vi "Main.vi"(10 "Monedas Sub Panel":refnum<vi>, 11 "Module Admin":refnum<class "Delacor_lib_QMH_Module Admin.lvclass">) -> ()   [LabVIEW 2020, in "Monedas.lvlib"]
doc: "This template is based off of the Queued Message Handler design pattern and the Queued Message Handler project template that ships with LabVIEW.\n\nThe main difference is that the queue is private to this module and communication between modules is performed via Broadcast and Request events.\n\nRequest events are wrapped in public API methods and are handled in the Event Handling Loop (EHL) of this VI. Any module can register for Broadcast events sent by this module. The EHL generates messages based on user interface actions.\n\nThe Message Handling Loop (MHL) processes messages generated by the EHL, or by other messages. The messages are string values, so new messages can be added easily to the Message Cases case structure in the MHL. Each message cluster can also provide an optional value for Message Data, which is a variant that can be converted to whatever message-specific data is required.\n_____\nBased on Delacor QMH Project Template 5.0.0.82."
uses:
  Monedas.lvlib
  <vilib>/Delacor/Delacor QMH/Libraries/Module Admin_class/Delacor_lib_QMH_Module Admin.lvclass
  Module Data--cluster.ctl
  Stop Argument--cluster.ctl
  <vilib>/Delacor/Delacor QMH/Libraries/Message Queue_class/Delacor_lib_QMH_Message Queue.lvclass/Delacor_lib_QMH_Message Queue.ctl
  Set Monedas Argument--cluster.ctl
  Producto Comprado Argument--cluster.ctl
  <vilib>/Delacor/Delacor QMH/Libraries/Module Admin_class/Delacor_lib_QMH_Module Admin.lvclass/Delacor_lib_QMH_Module Admin.ctl
  <vilib>/Delacor/Delacor QMH/Libraries/Message Queue_class/Delacor_lib_QMH_Enqueue Message (Single).vi
  <vilib>/Delacor/Delacor QMH/Libraries/Module Admin_class/Delacor_lib_QMH_Get External Launch.vi
  <vilib>/Utility/error.llb/Error Cluster From Error Code.vi
  <vilib>/ErrorRing/Error Ring.xnode
  <vilib>/Delacor/Delacor QMH/Libraries/Message Queue_class/Delacor_lib_QMH_Message Queue.lvclass
  Mensajes/Mensajes.lvlib
  Productos/Productos.lvlib
panel:
  in  "Monedas":T1
  out "error out":errorcluster
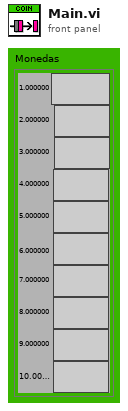
[diagram p1: front panel]
types:
  T1 = cluster{"Moneda 1":bool, "Moneda 2":bool, "Moneda 3":bool, "Moneda 4":bool, "Moneda 5":bool, "Moneda 6":bool, "Moneda 7":bool, "Moneda 8":bool, "Moneda 9":bool, "Moneda 10":bool}
  T2 = typedef "Monedas.lvlib/Request Events--cluster.ctl" = cluster{"Stop Module":refnum<user-event>, "Show Panel":refnum<user-event>, "Hide Panel":refnum<user-event>, "Get Module Execution Status":refnum<user-event>, "Show Diagram":refnum<user-event>, "Set Monedas":refnum<user-event>, "Producto Comprado":refnum<user-event>}
  T3 = typedef "Monedas.lvlib/Module Data--cluster.ctl" = cluster{"Status":string, "Array":cluster{"Numeric":dbl, "Boolean":bool}[], "Crédito":dbl}
  T4 = enum32{"invalid lock state", "Not Locked", "Locked (No Password)", "Password-protected"}
  T5 = typedef "Monedas.lvlib/Stop Argument--cluster.ctl" = cluster{"Origin":string, "Exit via Stop Module Req?":bool, "Wait for Module to stop?":bool}
  T6 = typedef "Monedas.lvlib/Set Monedas Argument--cluster.ctl" = cluster{"Monedas":cluster{"Numeric":dbl, "Boolean":bool}[]}
  T7 = typedef "Monedas.lvlib/Producto Comprado Argument--cluster.ctl" = cluster{"Numeric":dbl}
  T8 = enum32{"Invalid", "Standard", "Closed", "Hidden", "Minimized", "Maximized"}
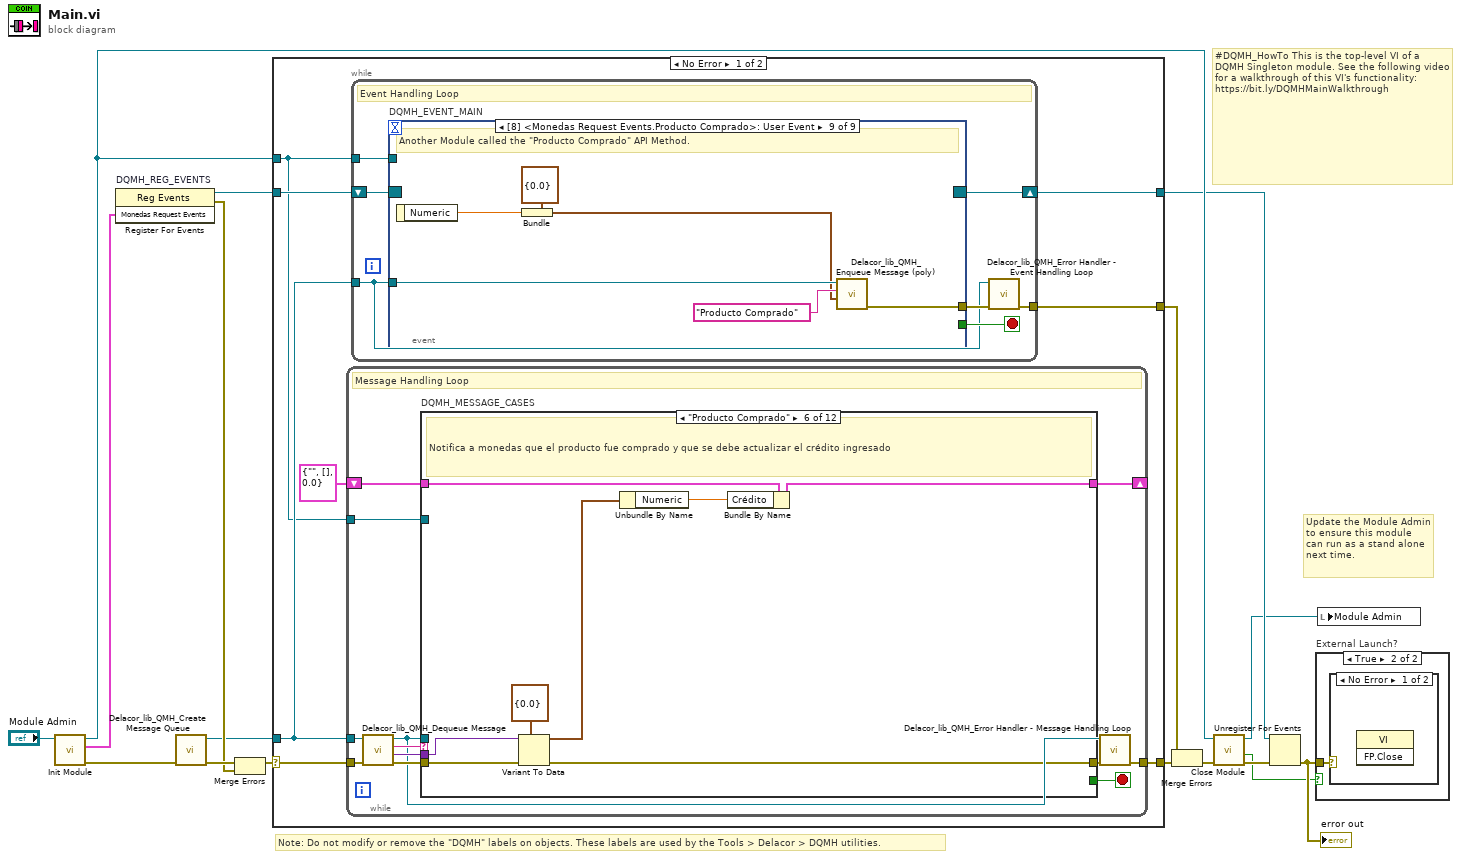
[diagram p0: block diagram]
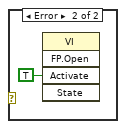
[diagram p3: hidden frame]
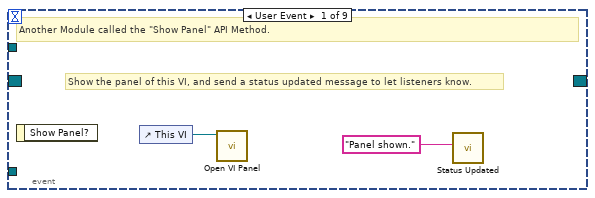
[diagram p4: hidden frame]
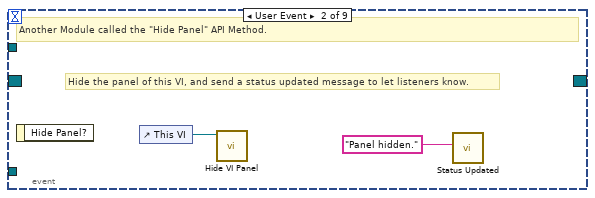
[diagram p5: hidden frame]
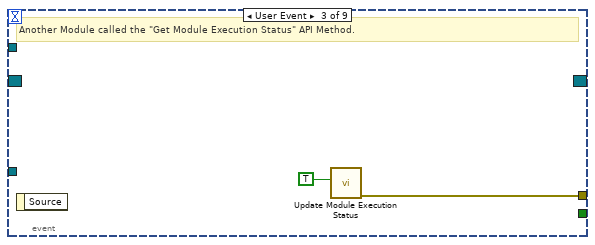
[diagram p6: hidden frame]
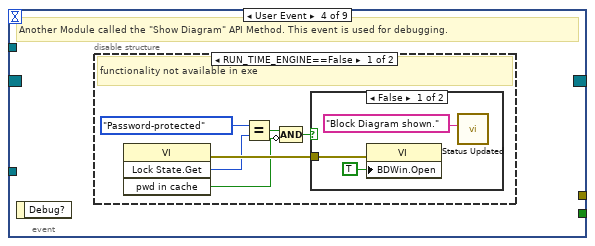
[diagram p7: hidden frame]
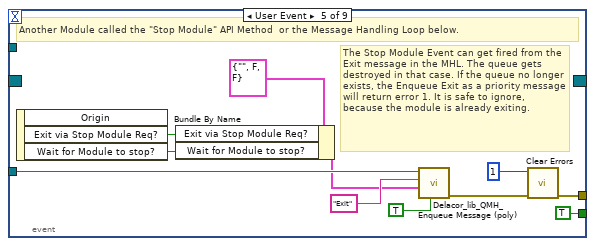
[diagram p10: hidden frame]
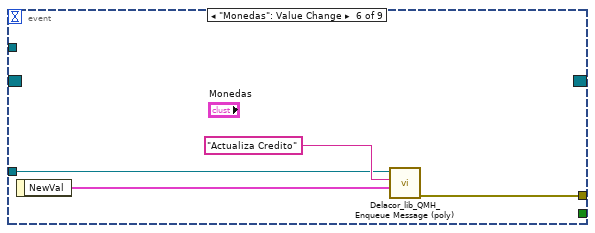
[diagram p11: hidden frame]
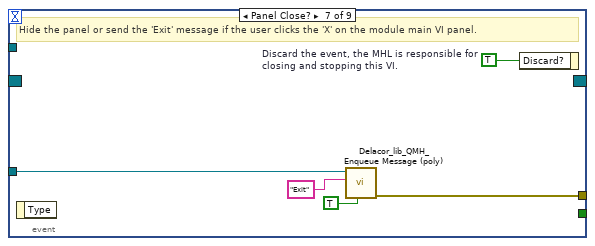
[diagram p12: hidden frame]
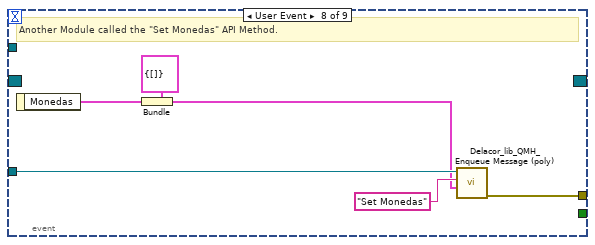
[diagram p13: hidden frame]
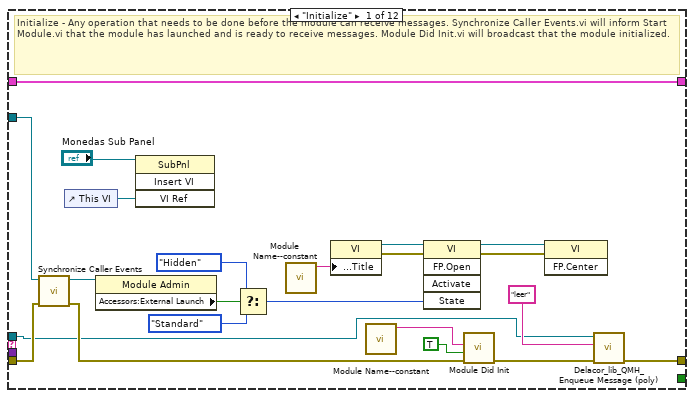
[diagram p14: hidden frame]
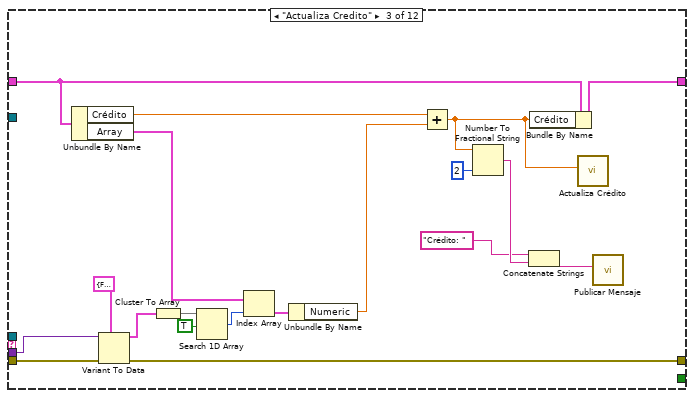
[diagram p16: hidden frame]
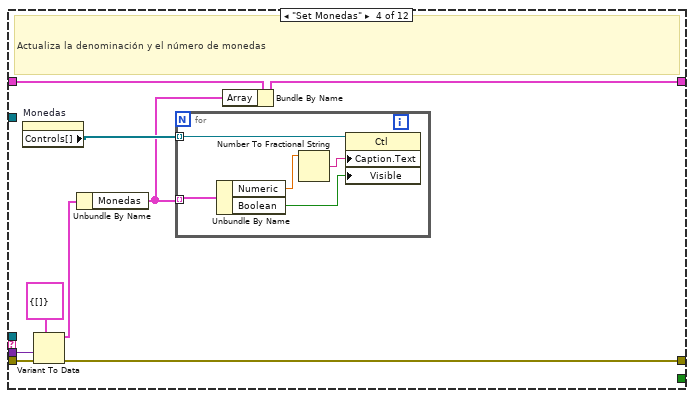
[diagram p17: hidden frame]
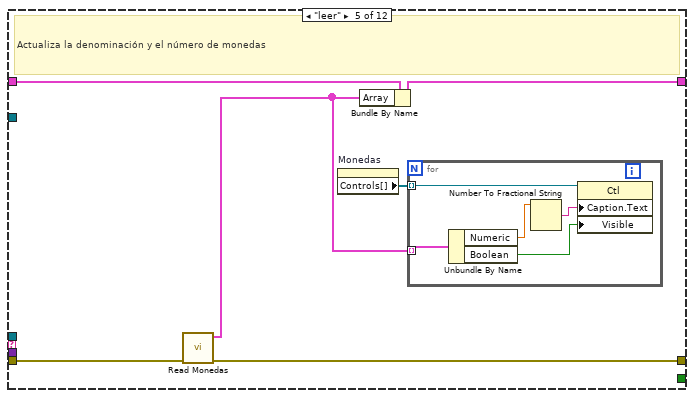
[diagram p18: hidden frame]
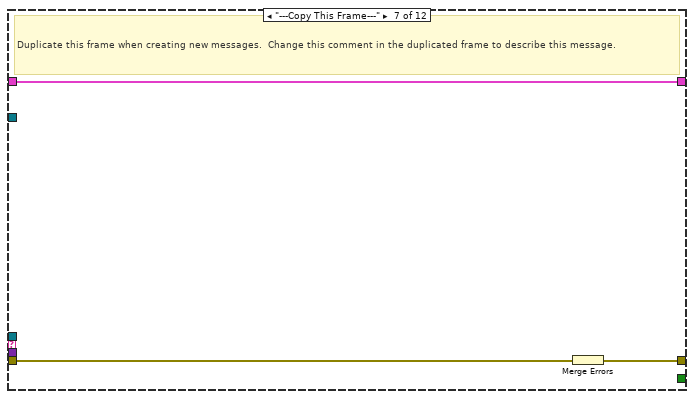
[diagram p19: hidden frame]
diagram:
  # "#DQMH_HowTo This is the top-level VI of a DQMH Singleton module. See the following video for a walkthrough of this VI's functionality: https://bit.ly/DQMHMainWalkthrough"
  # "Note: Do not modify or remove the \"DQMH\" labels on objects. These labels are used by the Tools > Delacor > DQMH utilities."
  # "Update the Module Admin to ensure this module can run as a stand alone next time."
  n1 = call "Init Module.vi"("Singleton Module Admin in"="Module Admin") -> ("error out"=w16:errorcluster, "Monedas Request Events"=w5:T2, "Singleton Module Admin out"=w8:refnum<class "Delacor_lib_QMH_Module Admin.lvclass">)  [unwired: 8 in]
  n2 = register-events "DQMH_REG_EVENTS"(w5) -> (reference out=w6:refnum<event-registration>, error out=w9:errorcluster)  [unwired: 2 in]
  n3 = call <vilib>:"Delacor_lib_QMH_Create Message Queue.vi"("error in (no error)"=w16) -> ("error out"=w11:errorcluster, "Message Queue"=w4:refnum<class "Delacor_lib_QMH_Message Queue.lvclass">)  [unwired: 9 in]
  n4 = Merge Errors(w11, w9) -> (w10:errorcluster)
  n5 = case shown="No Error" w10 {
    selector: w10 -> [w23 w233]
    tunnel: [w25 w232] -> w17
    tunnel: [w22 w238] -> w7
    tunnel: w6 -> [w20 w238]
    tunnel: w4 -> [w19 w231]
    tunnel: [w24 _] -> w14
    tunnel: w8 -> [w18 w234]
    frame No Error {
      n6 = while {
        tunnel: w19 -> [w82]
        shift-right: [w86] -> _
        shift-left: T3 {"Status"="", "Array"=[], "Crédito"=0.0} ("Data Cluster") -> [w87]
        tunnel: w23 -> [w90]
        tunnel: [w88] -> w25
        tunnel: w18 -> [w80]
        stop <- w85 stop-if-true
        # "Message Handling Loop"
        n7 = call-dynamic "Delacor_lib_QMH_Dequeue Message.vi"("error in (no error)"=w90, "Message Queue in"=w82) -> ("error out"=w89:errorcluster, "Message Data"=w83:variant, "Message"=w84:string, "Message Queue out"=w81:refnum<class "Delacor_lib_QMH_Message Queue.lvclass">)  [unwired: 6 in]
        n8 = case "DQMH_MESSAGE_CASES" shown="\"Producto Comprado\"" w84 {
          selector: w84 -> [_ _ _ _ _ _ _ _ _ _ _ w218]
          tunnel: w81 -> [w92 _ _ _ _ _ _ _ _ w188 w210 _]
          tunnel: w89 -> [w111 w115 w134 w143 w152 w167 w170 w172 w177 w195 w216 w220]
          tunnel: [w93 w115 w121 w135 w153 w165 w169 w172 w176 w191 w213 w221] -> w91
          tunnel: w87 -> [w101 w114 w127 w142 w154 w166 w168 w171 w174 w190 w209 w219]
          tunnel: [w101 w114 w124 w138 w151 w161 w168 w171 w174 w190 w209 w219] -> w86
          tunnel: [_ _ _ _ _ _ _ _ _ _ w208 _] -> w85
          tunnel: w83 -> [_ _ w133 w141 _ w164 _ _ _ w189 w207 _]
          tunnel: w80 -> [w102 _ _ _ _ _ _ _ _ w187 w202 _]
          frame "Initialize" {
            # "Initialize - Any operation that needs to be done before the module can receive messages. Synchronize Caller Events.vi will inform Start Module.vi that the module has launched and is ready to receive messages. Module Did Init.vi will broadcast that the module initialized."
            n9 = call "Synchronize Caller Events.vi"("error in (no error)"=w111, "Singleton Module Admin in"=w102) -> ("error out"=w110:errorcluster, "Singleton Module Admin out"=w98:refnum<class "Delacor_lib_QMH_Module Admin.lvclass">)  [unwired: 8 in]
            n10 = control-ref of="This VI"() -> (w96:refnum<vi>)
            n11 = property class="Module Admin"(reference=w98) -> ("Accessors:External Launch"=w106:bool)  [unwired: 1 in, 2 out]
            n12 = invoke class="SubPnl" method="Insert VI"(reference="Monedas Sub Panel", "VI Ref"=w96) -> ()  [unwired: 2 in, 4 out]
            n13 = Select(t=T8."Hidden" ("State"), s=w106, f=T8."Standard" ("State")) -> (s? t:f=w103:T8)
            n14 = call "Module Name--constant.vi"() -> ("Module Name"=w109:string)  [unwired: 11 in]
            n15 = property class="VI"("Front Panel.Title"=w109) -> (reference out=w108:refnum<vi>, error out=w113:errorcluster)  [unwired: 2 in]
            n16 = call "Module Name--constant.vi"() -> ("Module Name"=w99:string)  [unwired: 11 in]
            n17 = invoke class="VI" method="FP.Open"(reference=w108, error in=w113, "State"=w103) -> (reference out=w107:refnum<vi>, error out=w112:errorcluster)  [unwired: 2 in, 3 out]
            n18 = call "Module Did Init.vi"("error in (no error)"=w110, "Initialized?"=TRUE, "Origin"=w99) -> ("error out"=w94:errorcluster)  [unwired: 8 in]
            n19 = invoke class="VI" method="FP.Center"(reference=w107, error in=w112) -> ()  [unwired: 1 in, 3 out]
            n20 = call-poly <vilib>:"Delacor_lib_QMH_Enqueue Message (poly).vi"("error in (no error)"=w94, "Message"="leer", "Message Queue in"=w92) -> ("error out"=w93:errorcluster)  [unwired: 7 in, 1 out]
          }
          frame "--- Module Specific ---" {
            # "Separator -- The following cases handle messages specific to this Module."
          }
          frame "Actualiza Credito" {
            n21 = Unbundle By Name(w127) -> ("Crédito"=w122:dbl, "Array"=w126:cluster{"Numeric":dbl, "Boolean":bool}[])
            n22 = Variant To Data(error in=w134, type=T1 {"Moneda 1"=FALSE, "Moneda 2"=FALSE, "Moneda 3"=FALSE, "Moneda 4"=FALSE, "Moneda 5"=FALSE, "Moneda 6"=FALSE, "Moneda 7"=FALSE, "Moneda 8"=FALSE, "Moneda 9"=FALSE, "Moneda 10"=FALSE} ("Monedas"), Variant=w133) -> (data=w129:T1, error out=w121:errorcluster)
            n23 = Cluster To Array(cluster=w129) -> (array=w132:bool[])
            n24 = Search 1D Array(1D array=w132, element=TRUE) -> (index of element=w128:i32)  [unwired: 1 in]
            n25 = Index Array(array=w126, index=w128) -> (element=w125:cluster{"Numeric":dbl, "Boolean":bool})
            n26 = Unbundle By Name(w125) -> ("Numeric"=w123:dbl)
            n27 = Add(x=w122, y=w123) -> (x+y=w116:dbl)
            n28 = Number To Fractional String(number=w116, precision (6)=i16 2) -> (F-format string=w119:string)  [unwired: 2 in]
            n29 = Concatenate Strings("Crédito: " ("string"), w119) -> (w118:string)
            n30 = Bundle By Name(cluster=w127, "Crédito"=w116) -> (w124:T3)
            n31 = call "Actualiza Crédito.vi"("Crédito"=w116) -> ()  [unwired: 10 in, 1 out]
            n32 = call "Publicar Mensaje.vi"("Mensaje"=w118) -> ()  [unwired: 10 in, 1 out]
          }
          frame "Set Monedas" {
            # "Actualiza la denominación y el número de monedas"
            n33 = property on="Monedas" class="Clust"() -> ("Controls[]"=w137:refnum<vi>[])  [unwired: 2 in, 2 out]
            n34 = Variant To Data(error in=w143, type=T6 {"Monedas"=[]} ("Set Monedas Argument"), Variant=w141) -> (data=w139:T6, error out=w135:errorcluster)
            n35 = Unbundle By Name(w139) -> ("Monedas"=w136:cluster{"Numeric":dbl, "Boolean":bool}[])
            n36 = for {
              tunnel: w137 -> [w148] mode=indexing
              tunnel: w136 -> [w144] mode=indexing
              n37 = Unbundle By Name(w144) -> ("Numeric"=w146:dbl, "Boolean"=w145:bool)
              n38 = Number To Fractional String(number=w146) -> (F-format string=w147:string)  [unwired: 3 in]
              n39 = property class="Ctl"(reference=w148, "Caption.Text"=w147, "Visible"=w145) -> ()  [unwired: 1 in, 2 out]
            }
            n40 = Bundle By Name(cluster=w142, "Array"=w136) -> (w138:T3)
          }
          frame "leer" {
            # "Actualiza la denominación y el número de monedas"
            n41 = call "Read Monedas.vi"("error in (no error)"=w152) -> ("error out"=w153:errorcluster, "Array"=w150:cluster{"Numeric":dbl, "Boolean":bool}[])  [unwired: 9 in]
            n42 = property on="Monedas" class="Clust"() -> ("Controls[]"=w149:refnum<vi>[])  [unwired: 2 in, 2 out]
            n43 = Bundle By Name(cluster=w154, "Array"=w150) -> (w151:T3)
            n44 = for {
              tunnel: w149 -> [w159] mode=indexing
              tunnel: w150 -> [w157] mode=indexing
              n45 = Unbundle By Name(w157) -> ("Numeric"=w156:dbl, "Boolean"=w155:bool)
              n46 = Number To Fractional String(number=w156) -> (F-format string=w158:string)  [unwired: 3 in]
              n47 = property class="Ctl"(reference=w159, "Caption.Text"=w158, "Visible"=w155) -> ()  [unwired: 1 in, 2 out]
            }
          }
          frame "Producto Comprado" {
            # "Notifica a monedas que el producto fue comprado y que se debe actualizar el crédito ingresado"
            n48 = Variant To Data(error in=w167, type=T7 {"Numeric"=0.0} ("Producto Comprado Argument"), Variant=w164) -> (data=w162:T7, error out=w165:errorcluster)
            n49 = Unbundle By Name(w162) -> ("Numeric"=w160:dbl)
            n50 = Bundle By Name(cluster=w166, "Crédito"=w160) -> (w161:T3)
          }
          frame "---Copy This Frame---" {
            # "Duplicate this frame when creating new messages.  Change this comment in the duplicated frame to describe this message."
            n51 = Merge Errors(w170) -> (w169:errorcluster)
          }
          frame "--- Exit and Error Handling---" {
            # "Separator - The following cases handle errors and exit messages."
          }
          frame "Simulate MHL Error" {
            # "#DQMH_HowTo The 'Simulate MHL Error' button  illustrates how the MHL handles errors. This event is instructional in nature and can be removed."
            # "Simulate an error occurring at the MHL"
            n52 = call "Module Name--constant.vi"() -> ("Module Name"=w173:string)  [unwired: 11 in]
            n53 = xnode "Error Ring"("parameter 0"=w173) -> ("error out"=w175:errorcluster)
            n54 = Merge Errors(w177, w175) -> (w176:errorcluster)
          }
          frame "Error" {
            # "#CodeRecommended - If you ever change the name of this \"Error\" message, you'll need to update the name in the Check Loop Error.vi as well."
            # "#CodeRecommended - If the module is running in standalone mode (External Launch = FALSE), this code will pop up an error dialog and call the 'Exit' message if an error occurs. Add more fine-grained error handling here."
            # "Error - Check the error message data and respond accordingly. This message is sent by the \"Error Handler\" VIs at the end of each loop in this application."
            n55 = property class="Module Admin"(reference=w187) -> ("Accessors:External Launch"=w186:bool)  [unwired: 1 in, 2 out]
            n56 = Variant To Data(error in=w195, type=errorcluster {"status"=FALSE, "code"=0, "source"=""} ("error constant"), Variant=w189) -> (data=w196:errorcluster, error out=w193:errorcluster)
            n57 = call "Module Name--constant.vi"() -> ("Module Name"=w185:string)  [unwired: 11 in]
            n58 = call "Error Reported.vi"("Additional Information"=w185, "Error"=w196) -> ()  [unwired: 9 in, 1 out]
            n59 = case shown="False" w186 {
              tunnel: [w201 _] -> w192
              tunnel: w188 -> [w199 _]
              tunnel: w196 -> [w200 _]
              frame False {
                # "If the module is running standalone, then pop up an error dialog and call the \"Exit\" message."
                n60 = call <vilib>:"Simple Error Handler.vi"("error in (no error)"=w200) -> ()  [unwired: 4 in, 5 out]
                n61 = call-poly <vilib>:"Delacor_lib_QMH_Enqueue Message (poly).vi"("Priority Message? (F)"=TRUE, "Message"="Exit", "Message Queue in"=w199) -> ("error out"=w201:errorcluster)  [unwired: 7 in, 1 out]
              }
              frame True {
                # "If the module was launched externally, calling the Error Reported broadcast VI is the only action performed by the \"Error\" message. The module's caller can then process the error appropriately."
              }
            }
            n62 = Merge Errors(w193, w192) -> (w191:errorcluster)
            n63 = local write "error out"(w191) -> ()
          }
          frame "Exit" {
            w206 = 91  # 91: not all Exit messages will have an argument
            w208 = TRUE  # Stop the VI
            # "Release the message queue reference"
            # "#CodeNeeded - Add any required cleanup code here"
            # "Exit - Exit the application."
            n64 = Variant To Data(error in=w216, type=T5 {"Origin"="", "Exit via Stop Module Req?"=FALSE, "Wait for Module to stop?"=FALSE} ("Stop Argument"), Variant=w207) -> (data=w204:T5, error out=w212:errorcluster)
            n65 = call <vilib>:"Clear Errors.vi"("error in (no error)"=w212, "specific error code to clear (0: all)"=w206) -> ("error out"=w215:errorcluster)  [unwired: 4 in, 1 out]
            n66 = control-ref of="This VI"() -> (w203:refnum<vi>)
            n67 = call-dynamic "Delacor_lib_QMH_Release Message Queue.vi"("error in (no error)"=w215, "Message Queue"=w210) -> ("error out"=w214:errorcluster)  [unwired: 9 in]
            n68 = call "Handle Exit.vi"("Stop Argument"=w204, "Admin in"=w202, "VI reference"=w203) -> ("error out"=w211:errorcluster)  [unwired: 7 in, 1 out]
            n69 = Merge Errors(w214, w211) -> (w213:errorcluster)
          }
          frame Default {
            # "'Default' case only runs if there is a message that isn't defined in any of the other cases.  Output a programming error."
            n70 = call "Module Name--constant.vi"() -> ("Module Name"=w217:string)  [unwired: 11 in]
            n71 = xnode "Error Ring"("parameter 0"=w218, "parameter 1"=w217) -> ("error out"=w222:errorcluster)
            n72 = Merge Errors(w220, w222) -> (w221:errorcluster)
          }
        }
        n73 = call-dynamic "Delacor_lib_QMH_Error Handler - Message Handling Loop.vi"("error in (no error)"=w91, "Message Queue in"=w81) -> ("dup error in"=w88:errorcluster)  [unwired: 8 in, 1 out]
      }
      n74 = while {
        tunnel: w19 -> [w26]
        shift-right: [w29] -> w22
        shift-left: w20 -> [w30]
        tunnel: [w31] -> w24
        tunnel: w18 -> [w27]
        stop <- w28 stop-if-true
        # "Event Handling Loop"
        n75 = event "DQMH_EVENT_MAIN" shown="[8] <Monedas Request Events.Producto Comprado>: User Event" {
          selector: w30 -> [_ _ _ _ _ _ _ _ _]
          dyn-events: [_ _ _ _ _ _ _ _ _] -> w29
          timeout: _ -> [_ _ _ _ _ _ _ _ _]
          tunnel: [_ _ _ _ TRUE ("Discard?") _ _ _ _] -> w28
          tunnel: w26 -> [_ _ _ _ w54 w61 w65 w73 w79]
          tunnel: [_ _ w38 _ w57 w60 w67 w68 w74] -> w32
          tunnel: w27 -> [_ _ _ _ _ _ _ _ _]
          event User Event {
            # "Show the panel of this VI, and send a status updated message to let listeners know."
            # "Another Module called the \"Show Panel\" API Method."
            n76 = event-data() -> ()  [unwired: 1 in, 1 out]
            n77 = control-ref of="This VI"() -> (w34:refnum<vi>)
            n78 = call "Open VI Panel.vi"("VI"=w34) -> ()  [unwired: 10 in, 1 out]
            n79 = call "Status Updated.vi"("Status"="Panel shown." ("format string")) -> ()  [unwired: 10 in, 1 out]
          }
          event User Event {
            # "Hide the panel of this VI, and send a status updated message to let listeners know."
            # "Another Module called the \"Hide Panel\" API Method."
            n80 = event-data() -> ()  [unwired: 1 in, 1 out]
            n81 = control-ref of="This VI"() -> (w36:refnum<vi>)
            n82 = call "Hide VI Panel.vi"("VI"=w36) -> ()  [unwired: 10 in, 1 out]
            n83 = call "Status Updated.vi"("Status"="Panel hidden." ("format string")) -> ()  [unwired: 10 in, 1 out]
          }
          event User Event {
            # "Another Module called the \"Get Module Execution Status\" API Method."
            n84 = event-data() -> ()  [unwired: 1 in, 1 out]
            n85 = call "Update Module Execution Status.vi"("Running?"=TRUE) -> ("error out"=w38:errorcluster)  [unwired: 10 in]
          }
          event User Event {
            # "Another Module called the \"Show Diagram\" API Method. This event is used for debugging."
            n86 = event-data() -> ()  [unwired: 1 in, 1 out]
            n87 = disable-structure shown="RUN_TIME_ENGINE==False" {
              frame condition #0 (active) {
                # "functionality not available in exe"
                n88 = invoke class="VI" method="Lock State.Get"() -> (error out=w44:errorcluster, "Get Lock State"=w43:T4, "pwd in cache"=w40:bool)  [unwired: 4 in, 1 out]
                n89 = Equal?(x=T4."Password-protected", y=w43) -> (x = y?=w41:bool)
                n90 = Compound Arithmetic op=AND(w41, invert w40) -> (w39:bool)
                n91 = case shown="False" w39 {
                  tunnel: w44 -> [w47 _]
                  frame False {
                    n92 = property class="VI"(error in=w47, "BDWin.Open"=TRUE ("Block Diagram Window:Open")) -> ()  [unwired: 1 in, 2 out]
                    n93 = call "Status Updated.vi"("Status"="Block Diagram shown." ("format string")) -> ()  [unwired: 10 in, 1 out]
                  }
                  frame True {
                    # "Password-protected VI, and the password is not in the cache. Do not show the diagram."
                  }
                }
              }
              frame condition #1 {
              }
            }
          }
          event User Event {
            # "The Stop Module Event can get fired from the Exit message in the MHL. The queue gets destroyed in that case. If the queue no longer exists, the Enqueue Exit as a priority message will return error 1. It is safe to ignore, because the module is already exiting."
            # "Another Module called the \"Stop Module\" API Method  or the Message Handling Loop below."
            n94 = event-data() -> ("Exit via Stop Module Req?"=w50:bool, "Wait for Module to stop?"=w49:bool)  [unwired: 1 in, 1 out]
            n95 = Bundle By Name(cluster=T5 {"Origin"="", "Exit via Stop Module Req?"=FALSE, "Wait for Module to stop?"=FALSE} ("Stop Argument"), "Exit via Stop Module Req?"=w50, "Wait for Module to stop?"=w49) -> (w48:T5)
            n96 = call-poly <vilib>:"Delacor_lib_QMH_Enqueue Message (poly).vi"("Priority Message? (F)"=TRUE, "Message Data"=w48, "Message"="Exit", "Message Queue in"=w54) -> ("error out"=w58:errorcluster)  [unwired: 6 in, 1 out]
            n97 = call <vilib>:"Clear Errors.vi"("error in (no error)"=w58, "specific error code to clear (0: all)"=1) -> ("error out"=w57:errorcluster)  [unwired: 4 in, 1 out]
          }
          event "Monedas": Value Change {
            n98 = event-data() -> ("NewVal"=w59:T1)  [unwired: 1 in]
            n99 = call-poly <vilib>:"Delacor_lib_QMH_Enqueue Message (poly).vi"("Message Data"=w59, "Message"="Actualiza Credito", "Message Queue in"=w61) -> ("error out"=w60:errorcluster)  [unwired: 7 in, 1 out]
          }
          event Panel Close? {
            w66 = TRUE  # Discard the event, the MHL is responsible for closing and stopping this VI.
            # "Hide the panel or send the 'Exit' message if the user clicks the 'X' on the module main VI panel."
            n100 = event-data() -> ()  [unwired: 1 in, 1 out]
            n101 = call-poly <vilib>:"Delacor_lib_QMH_Enqueue Message (poly).vi"("Priority Message? (F)"=TRUE, "Message"="Exit", "Message Queue in"=w65) -> ("error out"=w67:errorcluster)  [unwired: 7 in, 1 out]
            n102 = event-data("Discard?"=w66) -> ()  [unwired: 1 in, 1 out]
          }
          event User Event {
            # "Another Module called the \"Set Monedas\" API Method."
            n103 = event-data() -> ("Monedas"=w69:cluster{"Numeric":dbl, "Boolean":bool}[])  [unwired: 1 in]
            n104 = Bundle(cluster=T6 {"Monedas"=[]} ("Set Monedas Argument"), "Monedas"=w69) -> (w70:T6)
            n105 = call-poly <vilib>:"Delacor_lib_QMH_Enqueue Message (poly).vi"("Message Data"=w70, "Message"="Set Monedas", "Message Queue in"=w73) -> ("error out"=w68:errorcluster)  [unwired: 7 in, 1 out]
          }
          event User Event {
            # "Another Module called the \"Producto Comprado\" API Method."
            n106 = event-data() -> ("Numeric"=w75:dbl)  [unwired: 1 in]
            n107 = Bundle(cluster=T7 {"Numeric"=0.0} ("Producto Comprado Argument"), "Numeric"=w75) -> (w76:T7)
            n108 = call-poly <vilib>:"Delacor_lib_QMH_Enqueue Message (poly).vi"("Message Data"=w76, "Message"="Producto Comprado", "Message Queue in"=w79) -> ("error out"=w74:errorcluster)  [unwired: 7 in, 1 out]
          }
        }
        n109 = call-dynamic "Delacor_lib_QMH_Error Handler - Event Handling Loop.vi"("error in (no error)"=w32, "Message Queue in"=w26) -> ("dup error in"=w31:errorcluster)  [unwired: 8 in, 1 out]
      }
    }
    frame Error {
      # "Synchronize Caller Events.vi will inform Start Module.vi that the module has launched and will let the code calling Start Module.vi register for broadcasts and would permit the caller receive the broadcast that an error occurred at launch time."
      n110 = call-dynamic "Delacor_lib_QMH_Release Message Queue.vi"("error in (no error)"=w233, "Message Queue"=w231) -> ("error out"=w232:errorcluster)  [unwired: 9 in]
      n111 = call "Synchronize Caller Events.vi"("Singleton Module Admin in"=w234) -> ("error out"=w239:errorcluster)  [unwired: 9 in, 1 out]
      n112 = call "Module Name--constant.vi"() -> ("Module Name"=w237:string)  [unwired: 11 in]
      n113 = Format Into String(format string="An error occurred during initialization. %s is no longer running.", w237) -> (resulting string=w235:string)  [unwired: 2 in, 1 out]
      n114 = Merge Errors(w232, w239) -> (w240:errorcluster)
      n115 = call "Error Reported.vi"("Additional Information"=w235, "Error"=w240) -> ()  [unwired: 9 in, 1 out]
    }
  }
  n116 = Merge Errors(w14, w17) -> (w13:errorcluster)
  n117 = call "Close Module.vi"("error in (no error)"=w13, "Module Admin in"=w8) -> ("error out"=w15:errorcluster, "External Launch"=w1:bool, "Module Admin out"=w2:refnum<class "Delacor_lib_QMH_Module Admin.lvclass">)  [unwired: 7 in]
  n118 = Unregister For Events(event registration refnum=w7, error in=w15) -> (error out=w12:errorcluster)
  "error out" <- w12
  n119 = case "External Launch?" shown="True" w1 {
    tunnel: w12 -> [_ w241]
    frame False {
    }
    frame True {
      n120 = case shown="No Error" w241 {
        frame No Error {
          n121 = invoke class="VI" method="FP.Close"() -> ()  [unwired: 3 in, 3 out]
        }
        frame Error {
          n122 = invoke class="VI" method="FP.Open"("Activate"=TRUE ("Activate?")) -> ()  [unwired: 4 in, 5 out]
        }
      }
    }
  }
  n123 = local write "Module Admin"(w2) -> ()
